vi "CloseClk.vi"(8 "error in (no error)":errorcluster, 10 "ClkName":string, 11 "PXI_MultiTrig in":refnum<class "PXI_MultiTrig.lvclass">) -> (0 "error out":errorcluster, 3 "PXI_MultiTrig out":refnum<class "PXI_MultiTrig.lvclass">)   [LabVIEW 2018, in "SyncPlugins.lvlib" / "PXI_MultiTrig.lvclass"]
uses:
  PXI_MultiTrig.lvclass
  PXI_MultiTrig.lvclass/PXI_MultiTrig.ctl
  Accessors/Write Clocks.vi
  Accessors/Read TimingSession.vi
  Accessors/Read RefClkSession.vi
  Accessors/Read Clocks.vi
  <vilib>/Utility/error.llb/Error Cluster From Error Code.vi
  <vilib>/ErrorRing/Error Ring.xnode
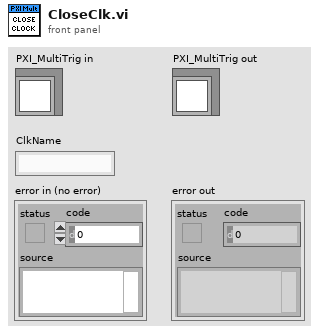
[diagram p1: front panel]
types:
  T1 = typedef "SyncPlugins.lvlib/PXI_MultiTrig.lvclass/clClocks.ctl" = cluster{"Name":string, "RefClk":string, "ClkTerminal":string, "Frequency":dbl, "DutyCycle":dbl, "ClkType":string, "Initiated":bool, "TrigTime":bool}
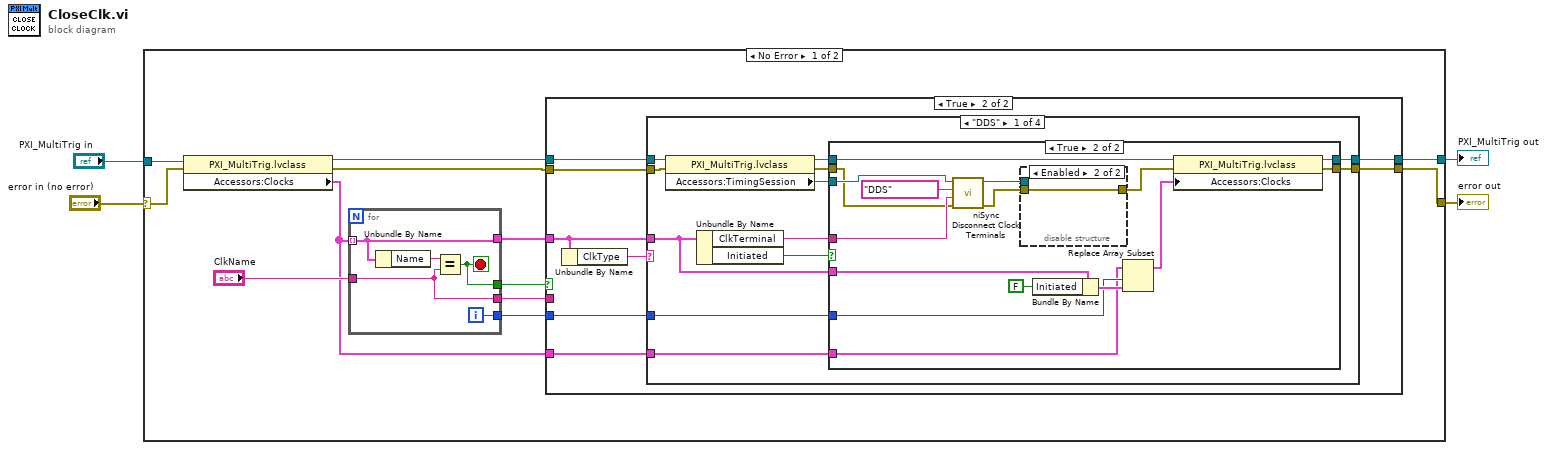
[diagram p0: block diagram]
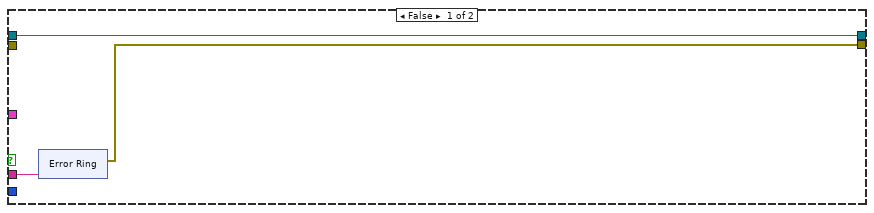
[diagram p2: hidden frame]
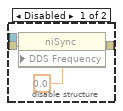
[diagram p4: hidden frame]
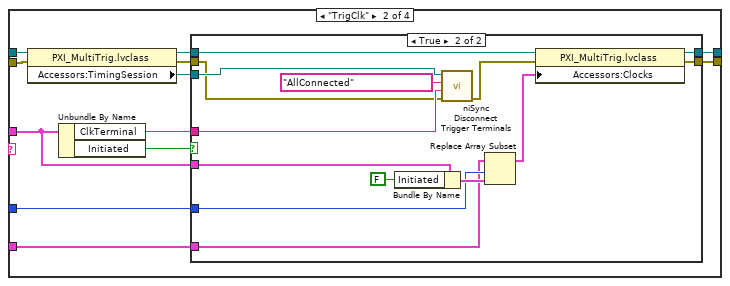
[diagram p5: hidden frame]
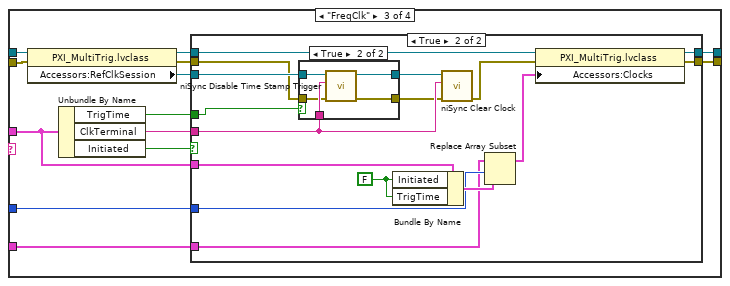
[diagram p7: hidden frame]
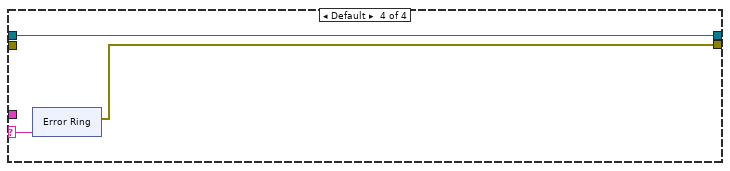
[diagram p10: hidden frame]
diagram:
  n1 = case shown="No Error" "error in (no error)" {
    selector: "error in (no error)" -> [w15 w151]
    tunnel: "PXI_MultiTrig in" -> [w16 w152]
    tunnel: [w6 w151] -> w2
    tunnel: [w5 w152] -> w1
    frame No Error {
      n2 = property class="PXI_MultiTrig.lvclass"(reference=w16, error in=w15) -> (reference out=w11:refnum<class "PXI_MultiTrig.lvclass">, error out=w7:errorcluster, "Accessors:Clocks"=w9:T1[])
      n3 = for {
        tunnel: w9 -> [w149] mode=indexing
        tunnel: "ClkName" -> [w147]
        tunnel: [w149] -> w10
        tunnel: [w148] -> w13
        tunnel: [w147] -> w12
        tunnel: [w146] -> w8
        i -> [w146]
        stop <- w148 stop-if-true
        n4 = Unbundle By Name(w149) -> ("Name"=w150:string)
        n5 = Equal?(x=w150, y=w147) -> (x = y?=w148:bool)
      }
      n6 = case shown="True" w13 {
        tunnel: w12 -> [w19 _]
        tunnel: w11 -> [w18 w33]
        tunnel: w10 -> [_ w32]
        tunnel: w9 -> [_ w30]
        tunnel: w8 -> [_ w31]
        tunnel: w7 -> [_ w29]
        tunnel: [w17 w28] -> w6
        tunnel: [w18 w27] -> w5
        frame False {
          n7 = xnode "Error Ring"("parameter 0"=w19) -> ("error out"=w17:errorcluster)
        }
        frame True {
          n8 = Unbundle By Name(w32) -> ("ClkType"=w34:string)
          n9 = case shown="\"DDS\"" w34 {
            selector: w34 -> [_ _ _ w138]
            tunnel: w33 -> [w45 w80 w109 w137]
            tunnel: w32 -> [w39 w74 w103 _]
            tunnel: w31 -> [w38 w73 w102 _]
            tunnel: w30 -> [w40 w75 w104 _]
            tunnel: w29 -> [w37 w72 w101 _]
            tunnel: [w36 w71 w100 w136] -> w28
            tunnel: [w35 w70 w99 w137] -> w27
            frame "DDS" {
              n10 = property class="PXI_MultiTrig.lvclass"(reference=w45, error in=w37) -> (reference out=w42:refnum<class "PXI_MultiTrig.lvclass">, error out=w41:errorcluster, "Accessors:TimingSession"=w44:refnum<k15>)
              n11 = Unbundle By Name(w39) -> ("ClkTerminal"=w46:string, "Initiated"=w43:bool)
              n12 = case shown="True" w43 {
                tunnel: w46 -> [_ w64]
                tunnel: w44 -> [_ w62]
                tunnel: w42 -> [w48 w53]
                tunnel: w41 -> [w47 w61]
                tunnel: w40 -> [_ w54]
                tunnel: w39 -> [_ w58]
                tunnel: w38 -> [_ w55]
                tunnel: [w48 w51] -> w35
                tunnel: [w47 w50] -> w36
                frame False {
                }
                frame True {
                  n13 = call <instrlib>:"niSync Disconnect Clock Terminals.vi"("error in (no error)"=w61, "destination terminal"=w64, "source terminal"="DDS", "instrument handle"=w62) -> ("error out"=w59:errorcluster, "instrument handle out"=w60:refnum<k15>)  [unwired: 6 in]
                  n14 = disable-structure shown="Enabled" {
                    disable-tunnel: w60 -> [w67 _]
                    disable-tunnel: w59 -> [w66 w69]
                    disable-tunnel: [w65 w69] -> w49
                    frame Disabled {
                      n15 = property class="niSync"(reference=w67, error in=w66, "DDS Frequency"=0.0 ("DDS Properties:DDS Frequency")) -> (error out=w65:errorcluster)  [unwired: 1 out]
                    }
                    frame Enabled {
                    }
                  }
                  n16 = Bundle By Name(cluster=w58, "Initiated"=FALSE) -> (w56:T1)
                  n17 = Replace Array Subset(array=w54, new element=w56, index=w55) -> (w52:T1[])
                  n18 = property class="PXI_MultiTrig.lvclass"(reference=w53, error in=w49, "Accessors:Clocks"=w52) -> (reference out=w51:refnum<class "PXI_MultiTrig.lvclass">, error out=w50:errorcluster)
                }
              }
            }
            frame "TrigClk" {
              n19 = property class="PXI_MultiTrig.lvclass"(reference=w80, error in=w72) -> (reference out=w77:refnum<class "PXI_MultiTrig.lvclass">, error out=w76:errorcluster, "Accessors:TimingSession"=w79:refnum<k15>)
              n20 = Unbundle By Name(w74) -> ("ClkTerminal"=w81:string, "Initiated"=w78:bool)
              n21 = case shown="True" w78 {
                tunnel: w81 -> [_ w97]
                tunnel: w79 -> [_ w96]
                tunnel: w77 -> [w83 w89]
                tunnel: w76 -> [w82 w95]
                tunnel: w75 -> [_ w90]
                tunnel: w74 -> [_ w94]
                tunnel: w73 -> [_ w91]
                tunnel: [w83 w87] -> w70
                tunnel: [w82 w86] -> w71
                frame False {
                }
                frame True {
                  n22 = Bundle By Name(cluster=w94, "Initiated"=FALSE) -> (w92:T1)
                  n23 = call <instrlib>:"niSync Disconnect Trigger Terminals.vi"("error in (no error)"=w95, "destination terminal"=w97, "source terminal"="AllConnected", "instrument handle"=w96) -> ("error out"=w84:errorcluster)  [unwired: 6 in, 1 out]
                  n24 = Replace Array Subset(array=w90, new element=w92, index=w91) -> (w88:T1[])
                  n25 = property class="PXI_MultiTrig.lvclass"(reference=w89, error in=w84, "Accessors:Clocks"=w88) -> (reference out=w87:refnum<class "PXI_MultiTrig.lvclass">, error out=w86:errorcluster)
                }
              }
            }
            frame "FreqClk" {
              n26 = property class="PXI_MultiTrig.lvclass"(reference=w109, error in=w101) -> (reference out=w106:refnum<class "PXI_MultiTrig.lvclass">, error out=w105:errorcluster, "Accessors:RefClkSession"=w108:refnum<k15>)
              n27 = Unbundle By Name(w103) -> ("TrigTime"=w98:bool, "ClkTerminal"=w110:string, "Initiated"=w107:bool)
              n28 = case shown="True" w107 {
                tunnel: w110 -> [_ w117]
                tunnel: w108 -> [_ w118]
                tunnel: w106 -> [w112 w124]
                tunnel: w105 -> [w111 w116]
                tunnel: w104 -> [_ w125]
                tunnel: w103 -> [_ w128]
                tunnel: w102 -> [_ w126]
                tunnel: [w112 w122] -> w99
                tunnel: [w111 w121] -> w100
                tunnel: w98 -> [_ w114]
                frame False {
                }
                frame True {
                  w113 = FALSE ("Initiated")
                  n29 = case shown="True" w114 {
                    tunnel: [w130 w135] -> w119
                    tunnel: w118 -> [w130 w134]
                    tunnel: w117 -> [_ w133]
                    tunnel: w116 -> [w129 w132]
                    tunnel: [w129 w131] -> w115
                    frame False {
                    }
                    frame True {
                      n30 = call <instrlib>:"niSync Disable Time Stamp Trigger.vi"("error in (no error)"=w132, "terminal"=w133, "instrument handle"=w134) -> ("error out"=w131:errorcluster, "instrument handle out"=w135:refnum<k15>)  [unwired: 6 in]
                    }
                  }
                  n31 = Bundle By Name(cluster=w128, "Initiated"=w113, "TrigTime"=w113) -> (w127:T1)
                  n32 = call <instrlib>:"niSync Clear Clock.vi"("error in (no error)"=w115, "terminal"=w117, "instrument handle"=w119) -> ("error out"=w120:errorcluster)  [unwired: 6 in, 1 out]
                  n33 = Replace Array Subset(array=w125, new element=w127, index=w126) -> (w123:T1[])
                  n34 = property class="PXI_MultiTrig.lvclass"(reference=w124, error in=w120, "Accessors:Clocks"=w123) -> (reference out=w122:refnum<class "PXI_MultiTrig.lvclass">, error out=w121:errorcluster)
                }
              }
            }
            frame Default {
              n35 = xnode "Error Ring"("parameter 0"=w138) -> ("error out"=w136:errorcluster)
            }
          }
        }
      }
    }
    frame Error {
    }
  }
  "error out" <- w2
  "PXI_MultiTrig out" <- w1
